vi "test.vi"() -> ()   [LabVIEW 2009]
uses:
  <vilib>/rvi/FXPMathLib/FxpSinAndCos/XNode/nifxpmath_SinAndCos.xnode
  <vilib>/rvi/FXPMathLib/FxpSinAndCos/subVIs/nifxpmath_SinAndCos_SimConfig.ctl
  <vilib>/rvi/FXPMathLib/FxpSinAndCos/simVIs/DllFxpSinAndCosTemp_sub.vi
  <vilib>/rvi/FXPMathLib/FxpPolarToRect/XNode/nifxpmath_PolarToRect.xnode
  <vilib>/rvi/FXPMathLib/FxpPolarToRect/subVIs/nifxpmath_PolarToRect_SimConfig.ctl
  <vilib>/rvi/FXPMathLib/FxpPolarToRect/simVIs/DllFxpPolarToRectTemp_sub.vi
panel:
  out "cos(x)":fxp<+/-,16,2> format="%.15g"
  out "sin(x)":fxp<+/-,16,2> format="%.15g"
  out "y":fxp<+/-,18,18>
  out "x":fxp<+/-,18,18>
  in  "phase (pi)":fxp<+,13,7> format="%.16g"
  in  "magnitude":fxp<+,16,16> format="%.15g"
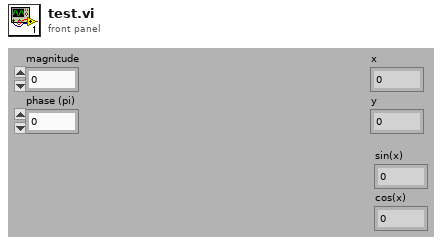
[diagram p1: front panel]
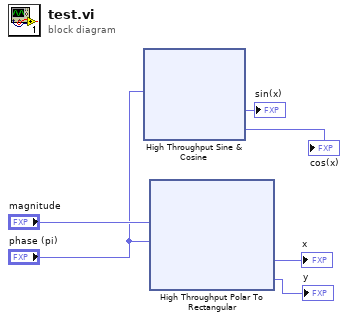
[diagram p0: block diagram]
diagram:
  n1 = xnode "High Throughput Sine & Cosine"("x (pi)"="phase (pi)") -> ("sin(x)"=→"sin(x)":fxp<+/-,16,2>, "cos(x)"=→"cos(x)":fxp<+/-,16,2>)
  n2 = xnode "High Throughput Polar To Rectangular"("magnitude"="magnitude", "phase (pi)"="phase (pi)") -> ("x"=→"x":fxp<+/-,18,18>, "y"=→"y":fxp<+/-,18,18>)
